vi "IntakeMain.vi"(0 "Control Mode":enum16{"Open", "Control"}(ring), 1 "Forwards":bool, 2 "Reverse":bool, 3 "Error In":errorcluster) -> (10 "Error Out":errorcluster)   [LabVIEW 2016]
uses:
  <vilib>/Rock Robotics/SystemInterfaces/DIO/FPGA_DIORelayChannel.ctl
  <vilib>/Rock Robotics/WPI/Relay/WPI_RelayDirection.ctl
  <vilib>/Rock Robotics/WPI/Relay/WPI_RelayValue.ctl
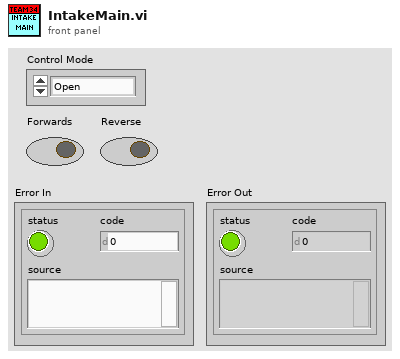
[diagram p1: front panel]
types:
  T1 = typedef "WPI_RelayDirection.ctl" = enum16{"Both directions", "Forward only", "Reverse only"}
  T2 = typedef "FPGA_DIORelayChannel.ctl" = enum8{"Relay 0", "Relay 1", "Relay 2", "Relay 3", "Invalid"}
  T3 = typedef "WPI_RelayValue.ctl" = enum16{"Off", "On", "Forward", "Reverse"}
  T4 = typedef "WPI_RelayDevRef.ctl" = cluster{"DevStatus":errorcluster, "Relay Channel":T2, "Relay Direction":T1}
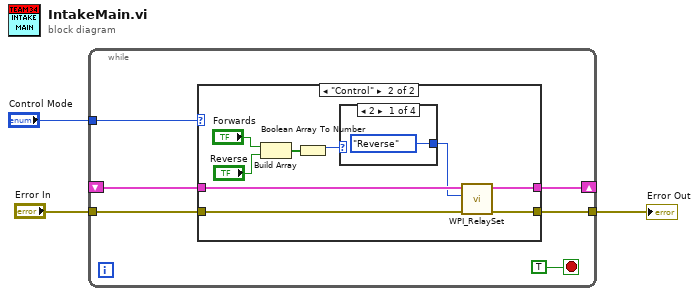
[diagram p0: block diagram]
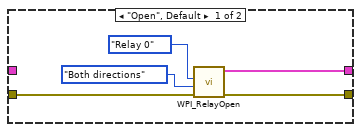
[diagram p2: hidden frame]
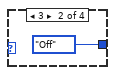
[diagram p3: hidden frame]
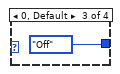
[diagram p4: hidden frame]
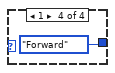
[diagram p5: hidden frame]
diagram:
  n1 = while {
    tunnel: "Control Mode" -> [w9]
    shift-right: [w7] -> _
    shift-left: _ -> [w6]
    tunnel: "Error In" -> [w5]
    tunnel: [w4] -> w1
    stop <- TRUE stop-if-true
    n2 = case shown="\"Control\"" w9 {
      tunnel: [w11 w16] -> w7
      tunnel: w6 -> [_ w18]
      tunnel: w5 -> [w10 w15]
      tunnel: [w10 w14] -> w4
      frame "Open", Default {
        n3 = call <vilib>:"WPI_RelayOpen.vi"("Relay Direction"=WPI_RelayDirection."Both directions", "Relay Channel"=FPGA_DIORelayChannel."Relay 0") -> ("RelayDevRef"=w11:T4)  [unwired: 8 in, 1 out]
      }
      frame "Control" {
        n4 = Build Array("Forwards", "Reverse") -> (w19:bool[])
        n5 = Boolean Array To Number(Boolean array=w19) -> (number=w20:u32)
        n6 = case shown="2" w20 {
          tunnel: [WPI_RelayValue."Reverse" ("RelayValue") WPI_RelayValue."Off" ("RelayValue") WPI_RelayValue."Off" ("RelayValue") WPI_RelayValue."Forward" ("RelayValue")] -> w17
          frame 2 {
          }
          frame 3 {
          }
          frame 0, Default {
          }
          frame 1 {
          }
        }
        n7 = call <vilib>:"WPI_RelaySet.vi"("error in (no error)"=w15, "RelayValue"=w17, "RelayDevRef"=w18) -> ("error out"=w14:errorcluster, "RelayDevRef"=w16:T4)  [unwired: 7 in]
      }
    }
  }
  "Error Out" <- w1
